vi "Get Channel By Name.vi"(8 "error in":errorcluster, 10 "Channel Name":string, 11 "Item in":refnum<class "Item.lvclass">) -> (0 "error out":errorcluster, 2 "Channel out":refnum<class "Channel.lvclass">, 3 "Item out":refnum<class "Item.lvclass">)   [LabVIEW 2024, in "Parser.lvlib" / "Channel.lvclass"]
uses:
  Channel.lvclass
  Channel.lvclass/Channel.ctl
  Item/Item.lvclass
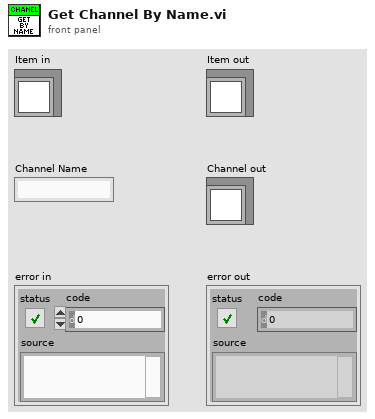
[diagram p1: front panel]
types:
  T1 = typedef "Parser.lvlib/Item.lvclass/Item Type.ctl" = enum16{"Channel", "Section"}
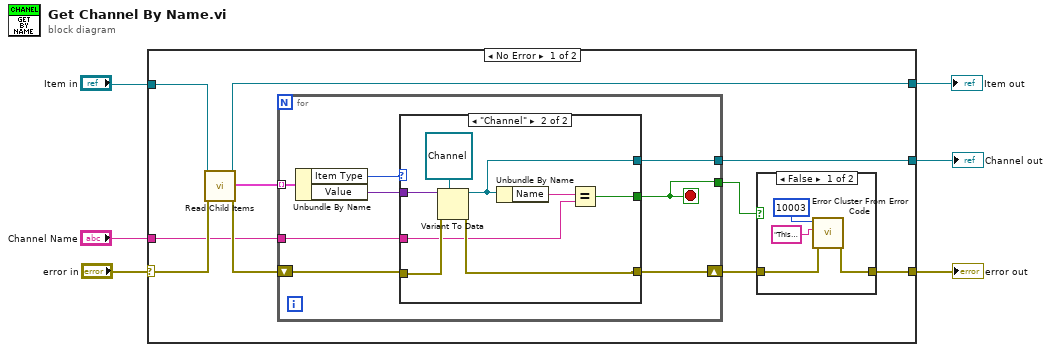
[diagram p0: block diagram]
diagram:
  n1 = case shown="No Error" "error in" {
    selector: "error in" -> [w13 w40]
    tunnel: [w16 w40] -> w6
    tunnel: "Channel Name" -> [w12 _]
    tunnel: "Item in" -> [w9 w39]
    tunnel: [w8 w39] -> w2
    tunnel: [w7 _] -> w1
    frame No Error {
      n2 = call "Read Child Items.vi"("error in"=w13, "Item in"=w9) -> ("error out"=w15:errorcluster, "Child Items"=w11:cluster{"Item Type":T1, "Value":variant}[], "Item out"=w8:refnum<class "Item.lvclass">)  [unwired: 7 in]
      n3 = for {
        tunnel: w11 -> [w27] mode=indexing
        tunnel: w12 -> [w24]
        shift-right: [w28] -> w14
        shift-left: w15 -> [w29]
        tunnel: [w23] -> w10
        tunnel: [w22] -> w7
        stop <- w23 stop-if-true
        n4 = Unbundle By Name(w27) -> ("Item Type"=w26:T1, "Value"=w25:variant)
        n5 = case shown="\"Channel\"" w26 {
          tunnel: w25 -> [_ w33]
          tunnel: w24 -> [_ w36]
          tunnel: [_ w35] -> w23
          tunnel: w29 -> [w30 w38]
          tunnel: [w30 w37] -> w28
          tunnel: [_ w31] -> w22
          frame Default {
          }
          frame "Channel" {
            n6 = Variant To Data(error in=w38, type=refnum<class "Channel.lvclass"> refnum ("Channel"), Variant=w33) -> (data=w31:refnum<class "Channel.lvclass">, error out=w37:errorcluster)
            n7 = Unbundle By Name(w31) -> ("Name"=w32:string)
            n8 = Equal?(x=w32, y=w36) -> (x = y?=w35:bool)
          }
        }
      }
      n9 = case shown="False" w10 {
        tunnel: w14 -> [w20 w21]
        tunnel: [w19 w21] -> w16
        frame False {
          n10 = call <vilib>:"Error Cluster From Error Code.vi"("error in (no error)"=w20, "error message (\"\")"="This Channel Does not exist.", "error code (0)"=10003) -> ("error out"=w19:errorcluster)  [unwired: 6 in]
        }
        frame True {
        }
      }
    }
    frame Error {
    }
  }
  "error out" <- w6
  "Item out" <- w2
  "Channel out" <- w1
